vi "Read Settings Cluster.vi"(8 "error in":errorcluster, 10 "variant":variant, 11 "Name":string) -> (0 "error out":errorcluster, 2 "Devicetype Variable \nData":string[][](array[string]))   [LabVIEW 2013]
doc: "This vi Read Settings cluster and update or add deviectype variable in Database for specified Device.\n\nInput\n1. Settings cluster\n2. DeviceName\n3. Error in\n\nOutput\n1. Devicetype Variable List\n2. Error Out"
uses:
  source/Device Driver/shared/numericVariable_TypeDef.ctl
  source/Device Driver/BaseDriver/BaseDriver.lvclass
panel:
  out "Data Name":string
  out "Array of VData":variant[](array[variant])
  # "(Taken for nested cluster names\neg Target cluster having x and y element \nthen name should be Target.X and Target.y)"
  # "Read variant input and parse Devicetype variable information from variant"
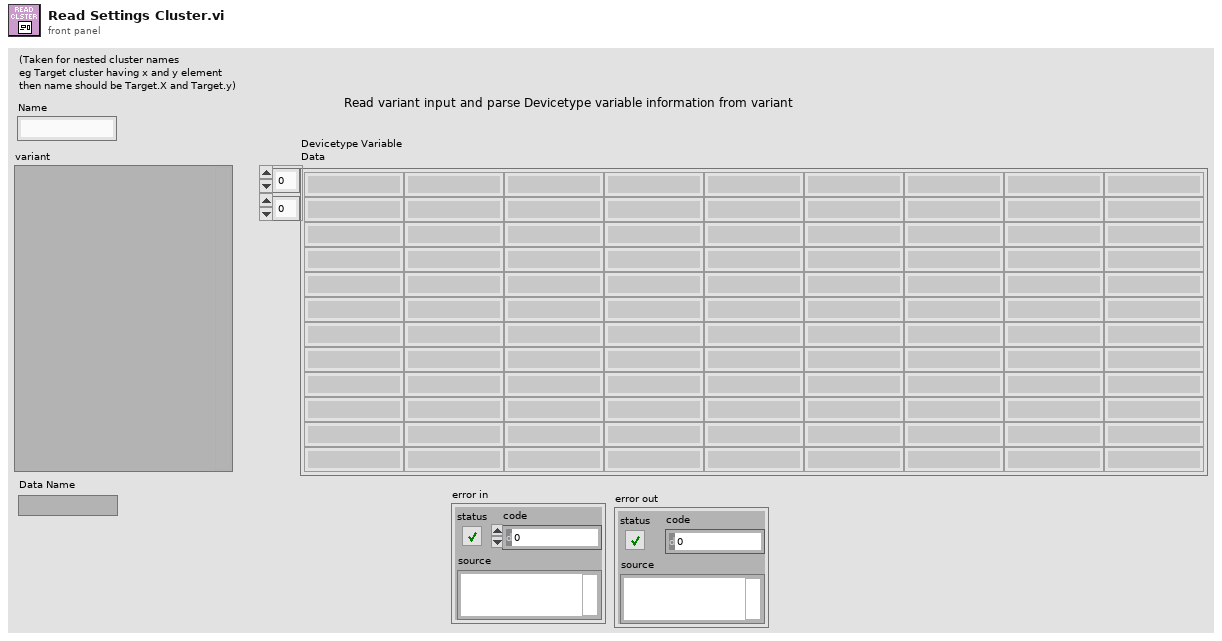
[diagram p1: front panel]
types:
  T1 = typedef "BaseDriver.lvclass/numericVariable_TypeDef.ctl" = cluster{"Value":dbl, "Min":dbl, "Max":dbl, "StepSize":dbl, "Tolerance":dbl, "ValueActual":dbl}
  T2 = cluster{"name":string, "value":string, "min":string, "max":string, "stepsize":string, "units":string, "variabletype":string, "tolerance":string, "valueactual":string}
  T3 = typedef "Type Descriptor Header__ogtk.ctl" = cluster{"length":u16, "private":u8, "type":T4, "# elements":u16}
  T4 = typedef "Type Descriptor Enumeration__ogtk.ctl" = enum8{"<Null>", "I8", "I16", "I32", "I64", "U8", "U16", "U32", "U64", "SGL", "DBL", "EXT", "CSG", "CDB", "CXT", "0x0F", "0x10", "0x11", "0x12", "0x13", "0x14", "Enum U8", "Enum U16", "Enum U32", "Enum U64", "SGL PQ", "DBL PQ", "EXT PQ", "CSG PQ", "CDB PQ", "CXT PQ", "0x1F", "0x20", "Boolean", "0x22", "0x23", "0x24", "0x25", "0x26", "0x27", "0x28", "0x29", "0x2A", "0x2B", "0x2C", "0x2D", "0x2E", "0x2F", "String", "0x31", "Path", "Pict", "0x34", "0x35", "0x36", "DAQ", "0x38", "0x39", "0x3A", "0x3B", "0x3C", "0x3D", "0x3E", "0x3F", "Array", "0x41", "0x42", "0x43", "0x44", "0x45", "0x46", "0x47", "0x48", "0x49", "0x4A", "0x4B", "0x4C", "0x4D", "0x4E", "0x4F", "Cluster", "0x51", "0x52", "Variant", "Waveform", "0x55", "0x56", "0x57", "0x58", "0x59", "0x5A", "0x5B", "0x5C", "0x5D", "0x5E", "0x5F", "0x60", "0x61", "0x62", "0x63", "0x64", "0x65", "0x66", "0x67", "0x68", "0x69", "0x6A", "0x6B", "0x6C", "0x6D", "0x6E", "0x6F", "Refnum"}
  T5 = typedef "Type Descriptor__ogtk.ctl" = i16[]
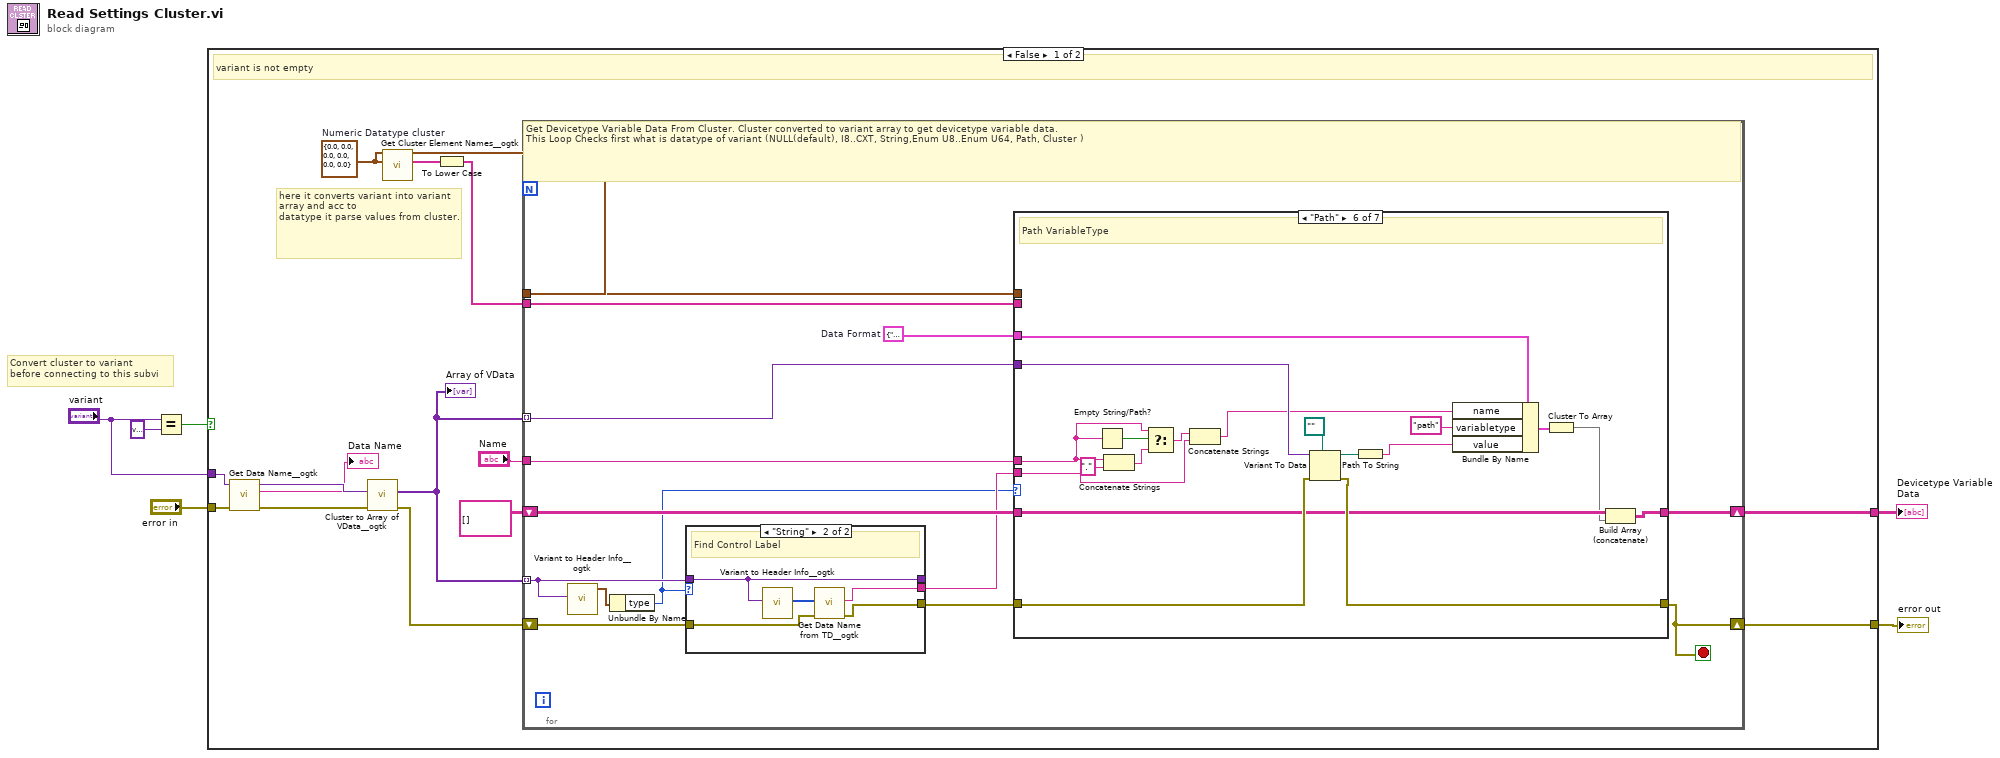
[diagram p0: block diagram]
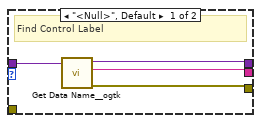
[diagram p2: hidden frame]
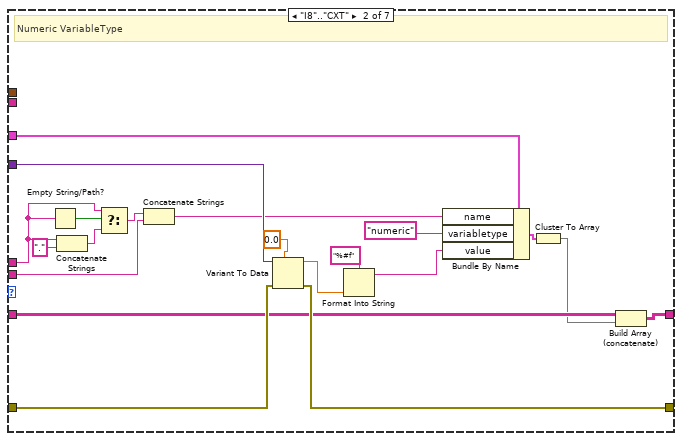
[diagram p4: hidden frame]
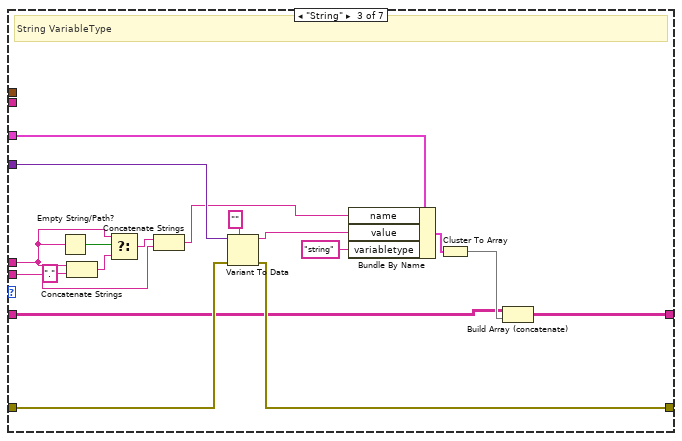
[diagram p5: hidden frame]
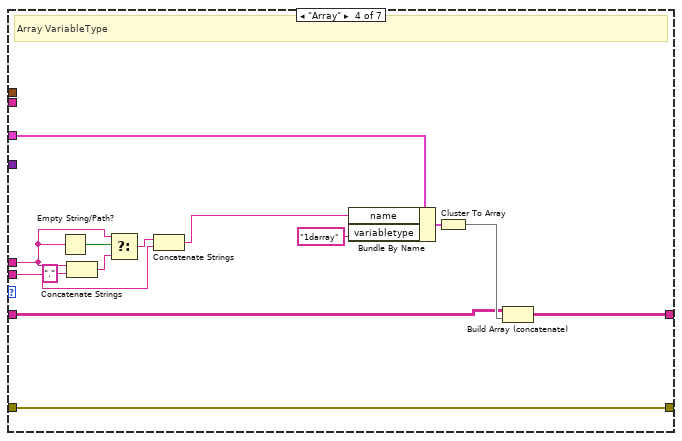
[diagram p6: hidden frame]
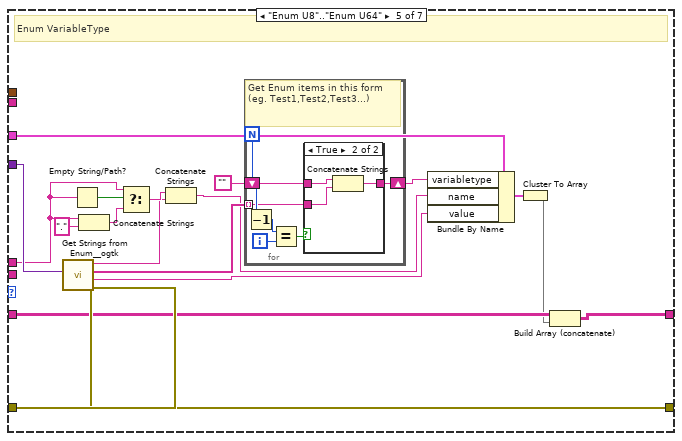
[diagram p7: hidden frame]
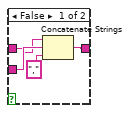
[diagram p8: hidden frame]
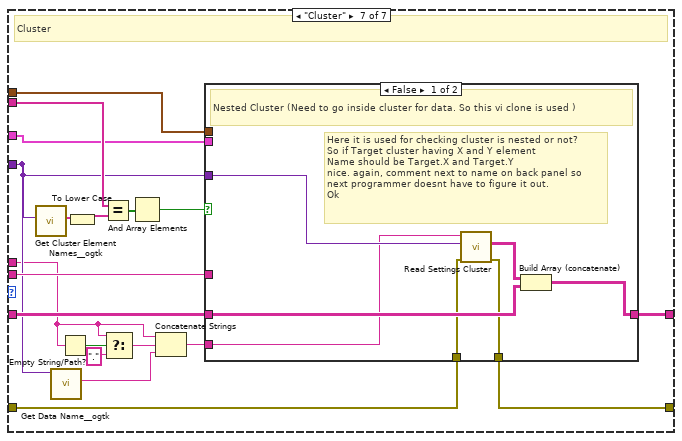
[diagram p9: hidden frame]
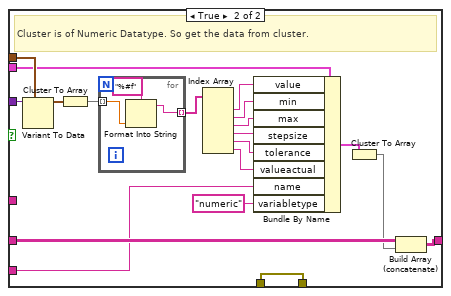
[diagram p10: hidden frame]
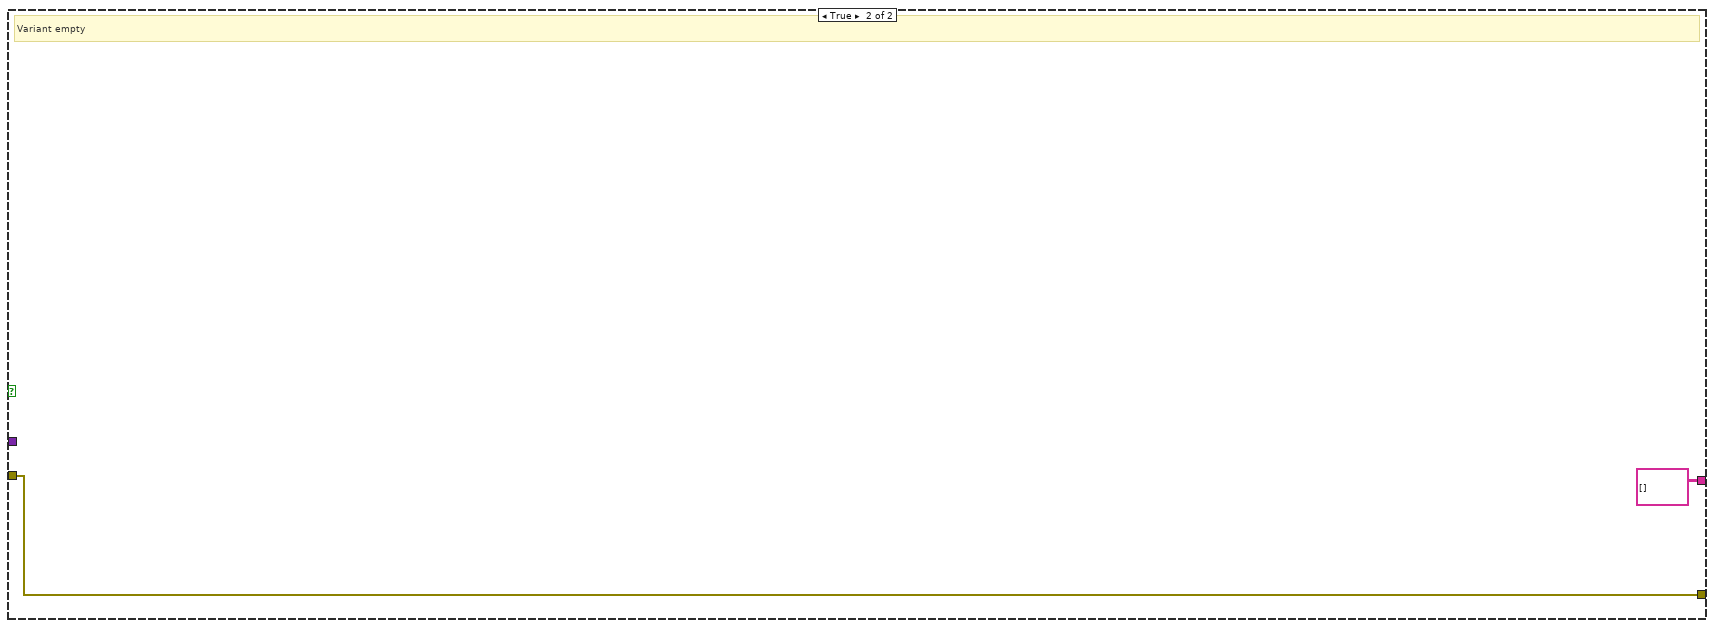
[diagram p11: hidden frame]
diagram:
  # "Convert cluster to variant \nbefore connecting to this subvi"
  n1 = Equal?(x="variant", y=variant) -> (x = y?=w4:bool)
  n2 = case shown="False" w4 {
    tunnel: "error in" -> [w16 w198]
    tunnel: "variant" -> [w9 _]
    tunnel: [w8 string[][] []] -> w2
    tunnel: [w7 w198] -> w1
    frame False {
      w11 = T1 {"Value"=0.0, "Min"=0.0, "Max"=0.0, "StepSize"=0.0, "Tolerance"=0.0, "ValueActual"=0.0}  # Numeric Datatype cluster
      # "here it converts variant into variant array and acc to \ndatatype it parse values from cluster."
      # "variant is not empty"
      n3 = call "Get Data Name__ogtk.vi"("error in (no error)"=w16, "Data"=w9) -> ("error out"=w18:errorcluster, "Data Name"=→"Data Name":string, "Data dup"=w20:variant)  [unwired: 7 in]
      n4 = call "Cluster to Array of VData__ogtk.vi"("error in (no error)"=w18, "Cluster"=w20) -> ("error out"=w17:errorcluster, "Array of VData"=w15:variant[])  [unwired: 8 in]
      "Array of VData" <- w15
      n5 = call "Get Cluster Element Names__ogtk.vi"("Cluster"=w11) -> ("Element Names"=w12:string[])  [unwired: 9 in, 1 out]
      n6 = To Lower Case(string=w12) -> (all lower case string=w10:string[])
      n7 = for {
        tunnel: w15 -> [w32] mode=indexing
        shift-right: [w33] -> w8
        shift-left: string[][] [] -> [w34]
        shift-right: [w23] -> w7
        shift-left: w17 -> [w31]
        tunnel: w15 -> [w25] mode=indexing
        tunnel: "Name" -> [w24]
        tunnel: w11 -> [w22]
        tunnel: w10 -> [w21]
        stop <- w23 stop-if-true
        w26 = T2 {"name"="", "value"="", "min"="", "max"="", "stepsize"="", "units"="", "variabletype"="", "tolerance"="", "valueactual"=""}  # Data Format
        # "Get Devicetype Variable Data From Cluster. Cluster converted to variant array to get devicetype variable data.\nThis Loop Checks first what is datatype of variant (NULL(default), I8..CXT, String,Enum U8..Enum U64, Path, Cluster )"
        n8 = call "Variant to Header Info__ogtk.vi"("Variant"=w32) -> ("Type Descriptor Header"=w27:T3)  [unwired: 3 in, 2 out]
        n9 = Unbundle By Name(w27) -> ("type"=w28:T4)
        n10 = case shown="\"String\"" w28 {
          tunnel: w31 -> [_ w43]
          tunnel: [w37 w42] -> w30
          tunnel: w32 -> [w38 w39]
          tunnel: [w36 w40] -> w29
          tunnel: [w35 w39] -> _
          frame "<Null>", Default {
            # "Find Control Label"
            n11 = call "Get Data Name__ogtk.vi"("Data"=w38) -> ("error out"=w37:errorcluster, "Data Name"=w36:string, "Data dup"=w35:variant)  [unwired: 8 in]
          }
          frame "String" {
            # "Find Control Label"
            n12 = call "Variant to Header Info__ogtk.vi"("Variant"=w39) -> ("Type Descriptor"=w41:T5)  [unwired: 3 in, 2 out]
            n13 = call "Get Data Name from TD__ogtk.vi"("error in (no error)"=w43, "Type Descriptor"=w41) -> ("error"=w42:errorcluster, "name"=w40:string)  [unwired: 8 in]
          }
        }
        n14 = case shown="\"Path\"" w28 {
          tunnel: w25 -> [_ w62 w83 _ w116 w146 w158]
          tunnel: w21 -> [_ _ _ _ _ _ w165]
          tunnel: w30 -> [w44 w60 w79 w84 w115 w145 w150]
          tunnel: [w44 w59 w77 w84 w114 w144 w151] -> w23
          tunnel: w34 -> [w45 w55 w74 w93 w107 w140 w160]
          tunnel: [w45 w53 w73 w92 w105 w138 w159] -> w33
          tunnel: w29 -> [_ w46 w66 w85 _ w131 w161]
          tunnel: w26 -> [_ w65 w81 w97 w111 w147 w162]
          tunnel: w22 -> [_ _ _ _ _ _ w163]
          tunnel: w24 -> [_ w50 w69 w88 w101 w134 w153]
          frame "<Null>", Default {
            # "NULL"
          }
          frame "I8".."CXT" {
            # "Numeric VariableType"
            n15 = Empty String/Path?(string/path=w50) -> (empty?=w52:bool)
            n16 = Concatenate Strings(w50, "." ("string")) -> (w51:string)
            n17 = Select(t=w50, s=w52, f=w51) -> (s? t:f=w47:string)
            n18 = Concatenate Strings(w47, w46) -> (w48:string)
            n19 = Variant To Data(error in=w60, type=0.0, Variant=w62) -> (data=w57:dbl, error out=w59:errorcluster)
            n20 = Format Into String(format string="%#f", w57) -> (resulting string=w56:string)  [unwired: 2 in, 1 out]
            n21 = Bundle By Name(cluster=w65, "name"=w48, "variabletype"="numeric", "value"=w56) -> (w63:T2)
            n22 = Cluster To Array(cluster=w63) -> (array=w54:string[])
            n23 = Build Array (concatenate)(w55, w54) -> (w53:string[][])
          }
          frame "String" {
            # "String VariableType"
            n24 = Empty String/Path?(string/path=w69) -> (empty?=w72:bool)
            n25 = Concatenate Strings(w69, "." ("string")) -> (w71:string)
            n26 = Select(t=w69, s=w72, f=w71) -> (s? t:f=w67:string)
            n27 = Concatenate Strings(w67, w66) -> (w68:string)
            n28 = Variant To Data(error in=w79, type="", Variant=w83) -> (data=w78:string, error out=w77:errorcluster)
            n29 = Bundle By Name(cluster=w81, "name"=w68, "value"=w78, "variabletype"="string") -> (w80:T2)
            n30 = Cluster To Array(cluster=w80) -> (array=w75:string[])
            n31 = Build Array (concatenate)(w74, w75) -> (w73:string[][])
          }
          frame "Array" {
            # "Array VariableType"
            n32 = Empty String/Path?(string/path=w88) -> (empty?=w91:bool)
            n33 = Concatenate Strings(w88, "." ("string")) -> (w90:string)
            n34 = Select(t=w88, s=w91, f=w90) -> (s? t:f=w86:string)
            n35 = Concatenate Strings(w86, w85) -> (w87:string)
            n36 = Bundle By Name(cluster=w97, "name"=w87, "variabletype"="1darray") -> (w96:T2)
            n37 = Cluster To Array(cluster=w96) -> (array=w94:string[])
            n38 = Build Array (concatenate)(w93, w94) -> (w92:string[][])
          }
          frame "Enum U8".."Enum U64" {
            # "Enum VariableType"
            n39 = call "Get Strings from Enum__ogtk.vi"("error in (no error)"=w115, "Enum"=w116) -> ("error out"=w114:errorcluster, "String Value"=w109:string, "Enum Strings"=w113:string[], "Enum Name"=w98:string)  [unwired: 6 in]
            n40 = Empty String/Path?(string/path=w101) -> (empty?=w104:bool)
            n41 = Concatenate Strings(w101, "." ("string")) -> (w103:string)
            n42 = Select(t=w101, s=w104, f=w103) -> (s? t:f=w99:string)
            n43 = Concatenate Strings(w99, w98) -> (w100:string)
            n44 = for {
              N -> [w123]
              tunnel: w113 -> [w118] mode=indexing
              shift-right: [w119] -> w110
              shift-left: "" -> [w117]
              i -> [w121]
              # "Get Enum items in this form (eg. Test1,Test2,Test3...)"
              n45 = Decrement(x=w123) -> (x-1=w122:i32)
              n46 = Equal?(x=w122, y=w121) -> (x = y?=w120:bool)
              n47 = case shown="True" w120 {
                tunnel: w118 -> [w126 w129]
                tunnel: [w125 w128] -> w119
                tunnel: w117 -> [w124 w130]
                frame False {
                  n48 = Concatenate Strings(w124, w126, ",") -> (w125:string)
                }
                frame True {
                  n49 = Concatenate Strings(w130, w129) -> (w128:string)
                }
              }
            }
            n50 = Bundle By Name(cluster=w111, "variabletype"=w110, "name"=w100, "value"=w109) -> (w108:T2)
            n51 = Cluster To Array(cluster=w108) -> (array=w106:string[])
            n52 = Build Array (concatenate)(w107, w106) -> (w105:string[][])
          }
          frame "Path" {
            # "Path VariableType"
            n53 = Empty String/Path?(string/path=w134) -> (empty?=w137:bool)
            n54 = Concatenate Strings(w134, "." ("string")) -> (w136:string)
            n55 = Select(t=w134, s=w137, f=w136) -> (s? t:f=w132:string)
            n56 = Concatenate Strings(w132, w131) -> (w133:string)
            n57 = Variant To Data(error in=w145, type=path "", Variant=w146) -> (data=w142:path, error out=w144:errorcluster)
            n58 = Path To String(path=w142) -> (string=w141:string)
            n59 = Bundle By Name(cluster=w147, "name"=w133, "variabletype"="path", "value"=w141) -> (w148:T2)
            n60 = Cluster To Array(cluster=w148) -> (array=w139:string[])
            n61 = Build Array (concatenate)(w140, w139) -> (w138:string[][])
          }
          frame "Cluster" {
            # "Cluster"
            n62 = call "Get Cluster Element Names__ogtk.vi"("Cluster"=w158) -> ("Element Names"=w168:string[])  [unwired: 9 in, 1 out]
            n63 = call "Get Data Name__ogtk.vi"("Data"=w158) -> ("Data Name"=w154:string)  [unwired: 8 in, 2 out]
            n64 = Empty String/Path?(string/path=w153) -> (empty?=w155:bool)
            n65 = To Lower Case(string=w168) -> (all lower case string=w167:string[])
            n66 = Equal?(x=w165, y=w167) -> (x = y?=w166:bool[])
            n67 = Select(t=w153, s=w155, f="." ("string")) -> (s? t:f=w157:string)
            n68 = And Array Elements(Boolean array=w166) -> (logical AND=w164:bool)
            n69 = Concatenate Strings(w153, w157, w154) -> (w152:string)
            n70 = case shown="False" w164 {
              tunnel: w163 -> [_ w192]
              tunnel: w158 -> [w175 w194]
              tunnel: w162 -> [_ w191]
              tunnel: w161 -> [_ _]
              tunnel: w160 -> [w174 w180]
              tunnel: [w173 w178] -> w159
              tunnel: w152 -> [w171 w177]
              tunnel: w150 -> [w170 w176]
              tunnel: [w169 w176] -> w151
              frame False {
                # "Here it is used for checking cluster is nested or not?\nSo if Target cluster having X and Y element \nName should be Target.X and Target.Y\nnice. again, comment next to name on back panel so\nnext programmer doesnt have to figure it out.\nOk"
                # "Nested Cluster (Need to go inside cluster for data. So this vi clone is used )"
                n71 = call "Read Settings Cluster.vi"("error in"=w170, "variant"=w175, "Name"=w171) -> ("error out"=w169:errorcluster, "Devicetype Variable \nData"=w172:string[][])  [unwired: 7 in]
                n72 = Build Array (concatenate)(w172, w174) -> (w173:string[][])
              }
              frame True {
                # "Cluster is of Numeric Datatype. So get the data from cluster."
                n73 = Variant To Data(type=w192, Variant=w194) -> (data=w182:T1)  [unwired: 1 in, 1 out]
                n74 = Cluster To Array(cluster=w182) -> (array=w193:dbl[])
                n75 = for {
                  tunnel: w193 -> [w197] mode=indexing
                  tunnel: [w196] -> w190 mode=indexing
                  n76 = Format Into String(format string="%#f", w197) -> (resulting string=w196:string)  [unwired: 2 in, 1 out]
                }
                n77 = Index Array(array=w190) -> (element #1=w189:string, element #2=w188:string, element #3=w187:string, element #4=w186:string, element #5=w185:string, element #6=w184:string)  [unwired: 6 in]
                n78 = Bundle By Name(cluster=w191, "value"=w189, "min"=w188, "max"=w187, "stepsize"=w186, "tolerance"=w185, "valueactual"=w184, "name"=w177, "variabletype"="numeric") -> (w181:T2)
                n79 = Cluster To Array(cluster=w181) -> (array=w179:string[])
                n80 = Build Array (concatenate)(w180, w179) -> (w178:string[][])
              }
            }
          }
        }
      }
    }
    frame True {
      # "Variant empty"
    }
  }
  "error out" <- w1
  "Devicetype Variable \nData" <- w2
